vi "Get_TEMPERATURE_Values_From_JSON.vi"(8 "Error In":errorcluster, 10 "utf-8 text":string="{\"rez\": 1289.454, \"status\": \"OK\", \"angle\": 89.616, \"temperature\": 7.252585, \"settings_nr\": 10, \"timestamp\": 1675537591.796923, \"resistance\": 1289.512, \"channel_nr\": 6, \"datetime\": \"2023-02-04T19:06:35.263978Z\", \"reactance\": 192510.068, \"magnitude\": 1289.483, \"status_flags\": [], \"imz\": 8.637}") -> (0 "Error Out":errorcluster, 1 "value":T1={"channel_nr"=6, "temperature"=7.252585, "resistance"=1289.512})   [LabVIEW 2017]
panel:
  in  "Cluster":T1
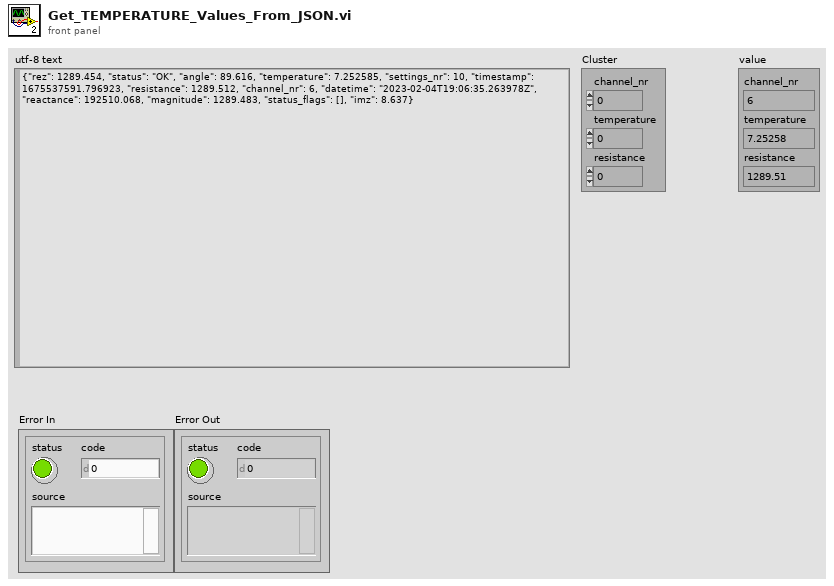
[diagram p1: front panel]
types:
  T1 = cluster{"channel_nr":i32, "temperature":dbl, "resistance":dbl}
  T2 = cluster{"id":i32, "name":string, "description":string}
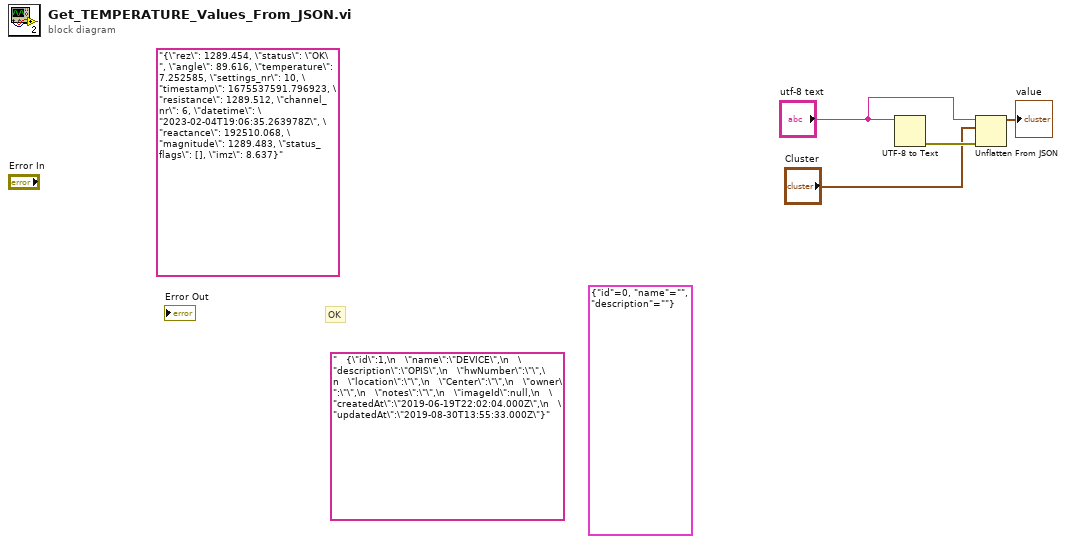
[diagram p0: block diagram]
diagram:
  (unwired) "{\"rez\": 1289.454, \"status\": \"OK\", \"angle\": 89.616, \"temperature\": 7.252585, \"settings_nr\": 10, \"timestamp\": 1675537591.796923, \"resistance\": 1289.512, \"channel_nr\": 6, \"datetime\": \"2023-02-04T19:06:35.263978Z\", \"reactance\": 192510.068, \"magnitude\": 1289.483, \"status_flags\": [], \"imz\": 8.637}" ("utf-8 text")
  (unwired) T2 {"id"=0, "name"="", "description"=""}
  (unwired) "   {\"id\":1,\n   \"name\":\"DEVICE\",\n   \"description\":\"OPIS\",\n   \"hwNumber\":\"\",\n   \"location\":\"\",\n   \"Center\":\"\",\n   \"owner\":\"\",\n   \"notes\":\"\",\n   \"imageId\":null,\n   \"createdAt\":\"2019-06-19T22:02:04.000Z\",\n   \"updatedAt\":\"2019-08-30T13:55:33.000Z\"}" ("utf-8 text")
  # "OK"
  n1 = UTF-8 to Text(11:"utf-8 text") -> (0:w4:errorcluster)  [unwired: 2 in, 1 out]
  n2 = Unflatten From JSON(JSON string="utf-8 text", type and defaults="Cluster", error in (no error)=w4) -> (value=→"value":T1)  [unwired: 4 in, 1 out]
